vi "SCP_Header_Bundle.vi"() -> (3 "Header Output":T1)   [LabVIEW 2018, in "SCP.lvlib"]
uses:
  SCP.lvlib
  Header_Type_Def.ctl
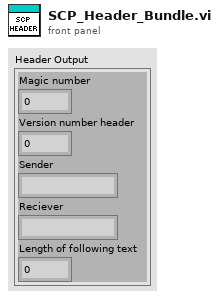
[diagram p1: front panel]
types:
  T1 = typedef "SCP.lvlib/Header_Type_Def.ctl" = cluster{"Magic number":u16, "Version number header":u16, "Sender":string, "Reciever":string, "Length of following text":i32}
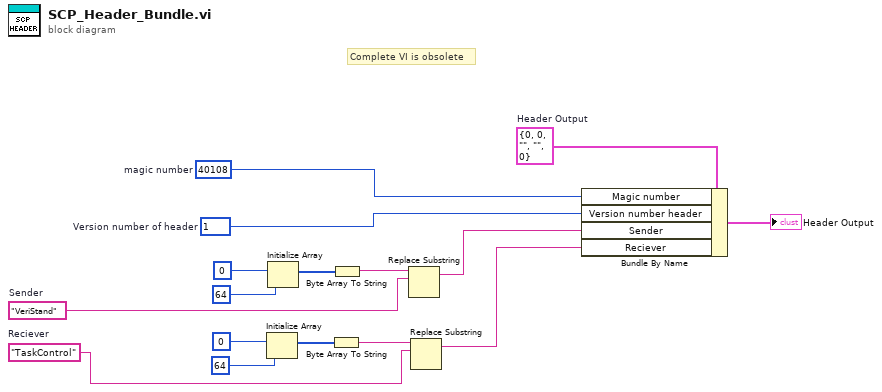
[diagram p0: block diagram]
diagram:
  w6 = T1 {"Magic number"=0, "Version number header"=0, "Sender"="", "Reciever"="", "Length of following text"=0}  # Header Output
  w16 = "TaskControl"  # Reciever
  w11 = "VeriStand"  # Sender
  w4 = u16 1  # Version number of header
  w5 = u16 40108  # magic number
  # "Complete VI is obsolete"
  n1 = Initialize Array(u8 0, 64 ("dimension size")) -> (w14:u8[])
  n2 = Initialize Array(u8 0, 64 ("dimension size")) -> (w8:u8[])
  n3 = Byte Array To String(unsigned byte array=w14) -> (string=w12:string)
  n4 = Byte Array To String(unsigned byte array=w8) -> (string=w10:string)
  n5 = Replace Substring(4:w11, 5:w10) -> (1:w3:string)  [unwired: 2 in, 1 out]
  n6 = Replace Substring(4:w16, 5:w12) -> (1:w2:string)  [unwired: 2 in, 1 out]
  n7 = Bundle By Name(cluster=w6, "Magic number"=w5, "Version number header"=w4, "Sender"=w3, "Reciever"=w2) -> (→"Header Output":T1)
